vi "Draw Mimic Image.vi"(11 "Mimic Data in":T1) -> (1 "Mimic Picture":picture)   [LabVIEW 2014, in "SeqLoop.lvlib" / "Mimico Display.lvlib"]
uses:
  Mimico Display.lvlib
  TypeDefs/Mimic Data.ctl
  TypeDefs/BG Image.ctl
  TypeDefs/mObject.ctl
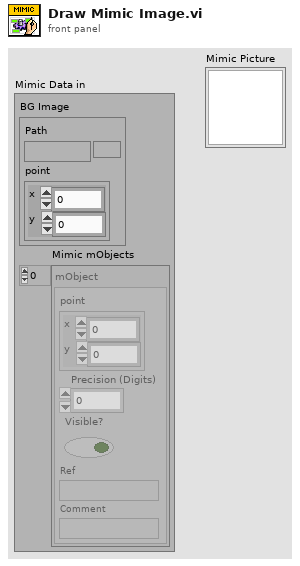
[diagram p1: front panel]
types:
  T1 = typedef "SeqLoop.lvlib/Mimico Display.lvlib/Mimic Data.ctl" = cluster{"BG Image":T2, "Mimic mObjects":T3[]}
  T2 = typedef "SeqLoop.lvlib/Mimico Display.lvlib/BG Image.ctl" = cluster{"Path":path, "point":cluster{"x":i16, "y":i16}}
  T3 = typedef "SeqLoop.lvlib/Mimico Display.lvlib/mObject.ctl" = cluster{"point":cluster{"x":i16, "y":i16}, "Precision (Digits)":i32, "Visible?":bool, "Ref":string, "Comment":string}
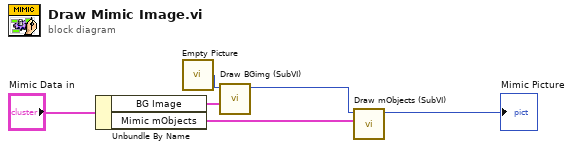
[diagram p0: block diagram]
diagram:
  n1 = Unbundle By Name("Mimic Data in") -> ("BG Image"=w3:T2, "Mimic mObjects"=w6:T3[])
  n2 = call "Empty Picture"() -> ("empty picture"=w1:picture)
  n3 = call "Draw BGimg (SubVI).vi"("BG Image"=w3, "picture in"=w1) -> ("picture out"=w2:picture)  [unwired: 9 in]
  n4 = call "Draw mObjects (SubVI).vi"("Mimic mObjects"=w6, "picture in"=w2) -> ("picture out"=→"Mimic Picture":picture)  [unwired: 9 in]
